vi "GetDataSourceFingerprint.vi"(8 "error in":errorcluster, 11 "Datawarehouse in":refnum<class "Datawarehouse.lvclass">) -> (0 "error out":errorcluster, 2 "DataSourceFingerprint":string, 3 "Datawarehouse out":refnum<class "Datawarehouse.lvclass">)   [LabVIEW 2021, in "ProligentXMLGenerator.lvlib" / "Datawarehouse.lvclass"]
doc: "The information contained in this attribute is used to protect the data warehouse from the\ninjection of the same file more than once. The rule is that all files that contain the\nsame fingerprint as a file that has already been processed successfully by the DIT will\nbe rejected.\n\nFor example, if the file contains information about a product unit, a good value for the\nfingerprint would be the product unit serial number followed by the generation date of the\nXSD.\n\nIf the attribute is ommited, the DIT will generate a random fingerprint. The result is\nthat it will now be possible to inject the same file more than once.\n\nThis value is limited to 448 charactesrs and must no be empty."
uses:
  Datawarehouse.lvclass
  Datawarehouse.lvclass/Datawarehouse.ctl
  Base/NonEmptyString_448/NonEmptyString_448.lvclass
  Base/Attribute/Attribute.lvclass
  C:/Projects/proligent-xml-generator-labview/src/ProligentXMLGenerator/Base/NonEmptyString/NonEmptyString.lvclass
  C:/Projects/proligent-xml-generator-labview/src/ProligentXMLGenerator/Base/String/String.lvclass
  C:/Projects/proligent-xml-generator-labview/src/ProligentXMLGenerator/Base/Attribute/Attribute.lvclass
  C:/Projects/proligent-xml-generator-labview/src/ProligentXMLGenerator/Base/NonEmptyString_448/NonEmptyString_448.lvclass
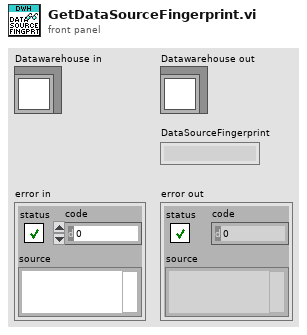
[diagram p1: front panel]
types:
  T1 = typedef "ProligentXMLGenerator.lvlib/Datawarehouse.lvclass/Data.ctl" = cluster{"DestinationFolder":path, "BaseFileName":string, "Document":refnum<k20>, "Defects":refnum<class "Defect.lvclass">[], "TopProcessRuns":refnum<class "ProcessRun.lvclass">[], "ProductUnits":refnum<class "ProductUnit.lvclass">[], "GenerationTime":refnum<class "DateTime.lvclass">, "DataSourceFingerprint":refnum<class "NonEmptyString_448.lvclass">, "IntegrationMetaData":refnum<class "NonEmptyString_2000.lvclass">, "TimeZoneInfoId":string}
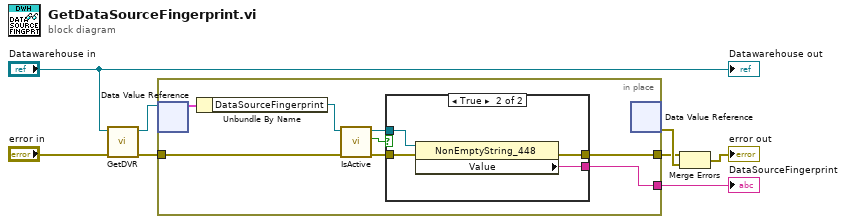
[diagram p0: block diagram]
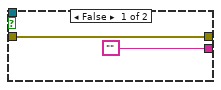
[diagram p2: hidden frame]
diagram:
  n1 = call "GetDVR.vi"("error in"="error in", "Datawarehouse"="Datawarehouse in") -> ("error out"=w5:errorcluster, "DVRReference"=w1:refnum<data-value>)  [unwired: 8 in]
  n2 = in-place "In Place Element Structure" {
    in-place-border: w5 -> [w12]
    in-place-border: [w15] -> w4
    in-place-border: [w14] -> w2
    n3 = in-place-dvr #1(w1) -> (w16:T1)  [unwired: 1 out]
    n4 = Unbundle By Name(w16) -> ("DataSourceFingerprint"=w13:refnum<class "NonEmptyString_448.lvclass">)
    n5 = call "IsActive.vi"("error in"=w12, "Attribute in"=w13) -> ("error out"=w9:errorcluster, "IsActive"=w10:bool, "Attribute in"=w11:refnum<class "NonEmptyString_448.lvclass">)  [unwired: 7 in]
    n6 = case shown="True" w10 {
      tunnel: [w18 w22] -> w15
      tunnel: ["" ("Empty String Constant") w21] -> w14
      tunnel: w11 -> [_ w20]
      tunnel: w9 -> [w18 w19]
      frame False {
      }
      frame True {
        n7 = property on="Property Node" class="NonEmptyString_448"(reference=w20, error in=w19) -> (error out=w22:errorcluster, "Value"=w21:string)  [unwired: 1 out]
      }
    }
    n8 = in-place-dvr #1() -> (w8:errorcluster)  [unwired: 1 in, 1 out]
  }
  "DataSourceFingerprint" <- w2
  n9 = Merge Errors(w4, w8) -> (→"error out":errorcluster)
  "Datawarehouse out" <- "Datawarehouse in"
